vi "LS100_READ.vi"(11 "Porta":refnum<visa-resource-name>="COM3") -> (0 "Visa Read Error Out":errorcluster, 2 "number (cd/m2)":dbl)   [LabVIEW 2017]
doc: "Simple demo program for Konica Minolta LS-100 and LS-110 control. LS-A12 serial cable required. 9 pin RS232 to USB converter, or add-in board, can be used for computers without serial header."
panel:
  out "Waveform Chart":dbl(graph)
  out "data string":string
  out "settings":string
  out "LS-100 error mssg":string
  in  "byte count":u32=17
  in  "write command":string="MES\r\n"
  out "read buffer":string
  in  "Continuous read":bool
  # "Measurement Loop will execute just once\nafter \"continuous read\" button is turned off.\nTurn off button and program should end normally"
  # "Make sure LS-100/110 is in\nC, computer control mode\nby Pressing F button while turning on"
  # "Konica Minolta LS-100/110\nusing LS-A12 2-way cable.\n\nNot for very old instruments using LS-A11\none-way cable."
  # "right click on graph to export data to clipboard or excel"
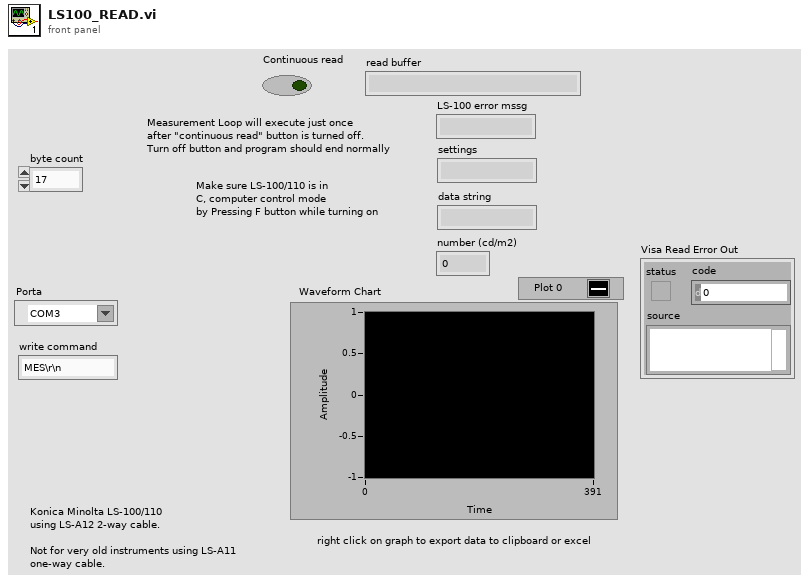
[diagram p1: front panel]
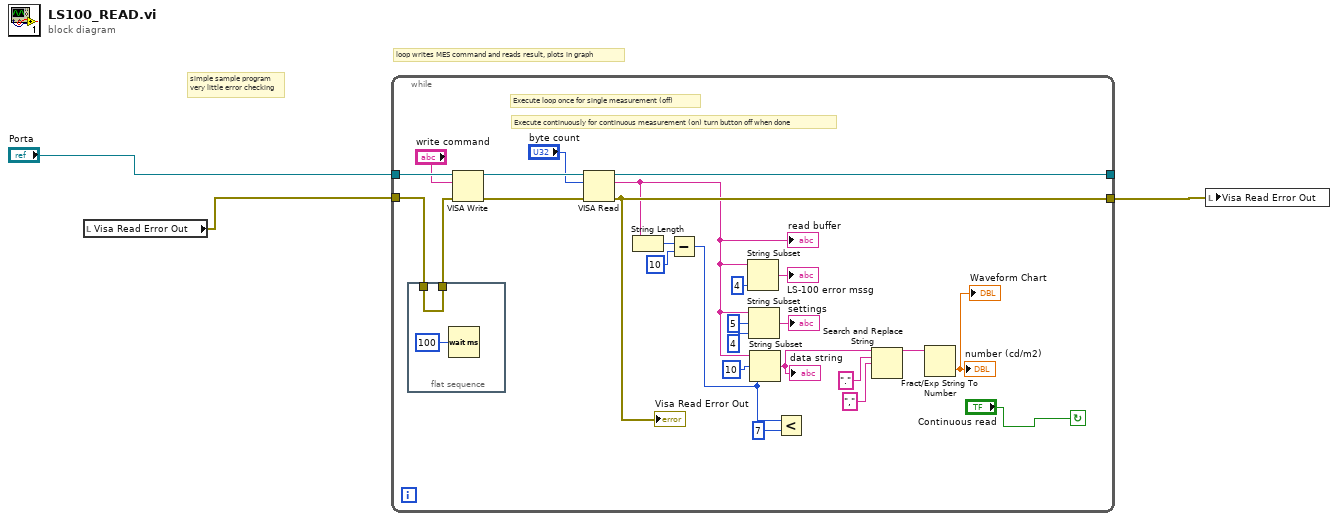
[diagram p0: block diagram]
diagram:
  # "loop writes MES command and reads result, plots in graph"
  # "simple sample program\nvery little error checking"
  n1 = local read "Visa Read Error Out"() -> (w2:errorcluster)
  n2 = while {
    tunnel: "Porta" -> [w28]
    tunnel: [w27] -> _
    tunnel: [w26] -> w1
    tunnel: w2 -> [w12]
    stop <- "Continuous read" continue-if-true
    # "Execute continuously for continuous measurement (on) turn button off when done"
    # "Execute loop once for single measurement (off)"
    n3 = flat-sequence {
      tunnel: w12 -> [w31]
      tunnel: [w31] -> w11
      frame #0 {
        n4 = Wait (ms)(milliseconds to wait=u32 100) -> ()  [unwired: 1 out]
      }
    }
    n5 = VISA Write(VISA resource name=w28, write buffer="write command", error in (no error)=w11) -> (VISA resource name out=w29:refnum<visa-resource-name>, error out=w25:errorcluster)  [unwired: 1 out]
    n6 = VISA Read(VISA resource name=w29, byte count="byte count", error in (no error)=w25) -> (VISA resource name out=w27:refnum<visa-resource-name>, read buffer=w14:string, error out=w26:errorcluster)  [unwired: 1 out]
    "read buffer" <- w14
    "Visa Read Error Out" <- w26
    n7 = String Length(string=w14) -> (length=w16:i32)
    n8 = Subtract(x=w16, y=10) -> (x-y=w5:i32)
    n9 = String Subset(string=w14, length (rest)=4 ("length (rest)")) -> (substring=→"LS-100 error mssg":string)  [unwired: 1 in]
    n10 = String Subset(string=w14, offset (0)=5, length (rest)=4 ("length (rest)")) -> (substring=→"settings":string)
    n11 = String Subset(string=w14, offset (0)=10, length (rest)=w5) -> (substring=w8:string)
    "data string" <- w8
    n12 = Less?(x=w5, y=7) -> ()  [unwired: 1 out]
    n13 = Search and Replace String(input string=w8, search string=".", replace string="," ("replace string (\"\")")) -> (result string=w7:string)  [unwired: 5 in, 3 out]
    n14 = Fract/Exp String To Number(string=w7) -> (number=→"number (cd/m2)" →"Waveform Chart":dbl)  [unwired: 3 in, 1 out]
  }
  n15 = local write "Visa Read Error Out"(w1) -> ()
